vi "Write File Path Control.vi"(8 "error in (no error)":errorcluster, 10 "Function Locations":path[](array[path]), 11 "Load Functions Message in":refnum<class "Find Functions On Disk Message.lvclass">) -> (0 "error out":errorcluster, 3 "Load Functions Message out":refnum<class "Find Functions On Disk Message.lvclass">)   [LabVIEW 2016, in "Controller Actor.lvlib" / "Find Functions On Disk Message.lvclass"]
uses:
  <userlib>/Common Components/Controller/Messages/Load Functions/Find Functions On Disk Message.lvclass
  <userlib>/Common Components/Controller/Messages/Load Functions/Find Functions On Disk Message.lvclass/Find Functions On Disk Message.ctl
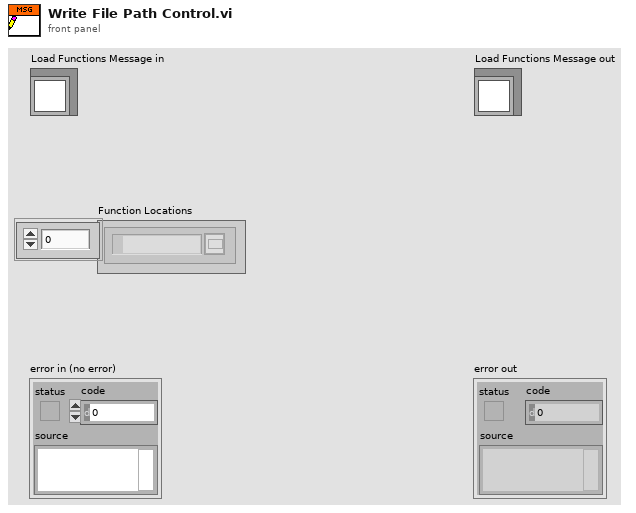
[diagram p1: front panel]
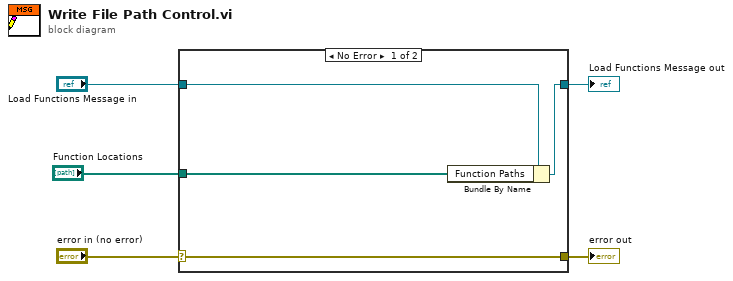
[diagram p0: block diagram]
diagram:
  n1 = case shown="No Error" "error in (no error)" {
    selector: "error in (no error)" -> [w9 w10]
    tunnel: [w9 w10] -> w4
    tunnel: [w7 w11] -> w2
    tunnel: "Load Functions Message in" -> [w8 w11]
    tunnel: "Function Locations" -> [w6 _]
    frame No Error {
      n2 = Bundle By Name(cluster=w8, "Function Paths"=w6) -> (w7:refnum<class "Find Functions On Disk Message.lvclass">)
    }
    frame Error {
    }
  }
  "error out" <- w4
  "Load Functions Message out" <- w2
